vi "Next Generation.vi"(11 "cells in":bool[][](array[boolean])=[[FALSE, FALSE, TRUE, FALSE, FALSE, FALSE, FALSE, FALSE, FALSE, FALSE, FALSE, FALSE, FALSE, FALSE, FALSE, FALSE], [FALSE, FALSE, FALSE, TRUE, TRUE, FALSE, FALSE, FALSE, FALSE, FALSE, FALSE, FALSE, FALSE, FALSE, FALSE, FALSE], [FALSE, FALSE, FALSE, FALSE, FALSE, FALSE, FALSE, FALSE, FALSE, FALSE, FALSE, FALSE, FALSE, FALSE, FALSE, FALSE], [FALSE, FALSE, FALSE, FALSE, FALSE, FALSE, FALSE, FALSE, FALSE, FALSE, FALSE, FALSE, FALSE, FALSE, FALSE, FALSE], [FALSE, FALSE, FALSE, FALSE, FALSE, FALSE, FALSE, FALSE, FALSE, FALSE, FALSE, FALSE, FALSE, FALSE, FALSE, FALSE], [FALSE, FALSE, FALSE, FALSE, FALSE, FALSE, FALSE, FALSE, FALSE, FALSE, FALSE, FALSE, FALSE, FALSE, FALSE, FALSE], [FALSE, FALSE, FALSE, FALSE, FALSE, FALSE, FALSE, TRUE, FALSE, FALSE, FALSE, FALSE, FALSE, FALSE, FALSE, FALSE], [FALSE, FALSE, FALSE, FALSE, FALSE, FALSE, FALSE, FALSE, FALSE, FALSE, FALSE, FALSE, FALSE, FALSE, FALSE, FALSE], [FALSE, FALSE, FALSE, FALSE, FALSE, FALSE, FALSE, FALSE, FALSE, FALSE, FALSE, FALSE, FALSE, FALSE, FALSE, FALSE], [FALSE, FALSE, FALSE, FALSE, FALSE, FALSE, FALSE, FALSE, FALSE, FALSE, FALSE, FALSE, FALSE, TRUE, FALSE, FALSE], [FALSE, FALSE, FALSE, FALSE, FALSE, FALSE, FALSE, FALSE, FALSE, FALSE, FALSE, FALSE, TRUE, TRUE, FALSE, FALSE], [FALSE, FALSE, FALSE, FALSE, FALSE, FALSE, FALSE, FALSE, FALSE, FALSE, FALSE, FALSE, FALSE, FALSE, TRUE, FALSE], [FALSE, FALSE, FALSE, FALSE, FALSE, FALSE, FALSE, FALSE, FALSE, FALSE, FALSE, FALSE, FALSE, FALSE, FALSE, TRUE]]) -> (1 "deaths":i32, 2 "births":i32, 3 "cells out":bool[][](array[boolean])=[[FALSE, FALSE, FALSE, TRUE, FALSE, FALSE, FALSE, FALSE, FALSE, FALSE, FALSE, FALSE, FALSE, FALSE, FALSE, FALSE], [FALSE, FALSE, FALSE, TRUE, FALSE, FALSE, FALSE, FALSE, FALSE, FALSE, FALSE, FALSE, FALSE, FALSE, FALSE, FALSE], [FALSE, FALSE, FALSE, FALSE, FALSE, FALSE, FALSE, FALSE, FALSE, FALSE, FALSE, FALSE, FALSE, FALSE, FALSE, FALSE], [FALSE, FALSE, FALSE, FALSE, FALSE, FALSE, FALSE, FALSE, FALSE, FALSE, FALSE, FALSE, FALSE, FALSE, FALSE, FALSE], [FALSE, FALSE, FALSE, FALSE, FALSE, FALSE, FALSE, FALSE, FALSE, FALSE, FALSE, FALSE, FALSE, FALSE, FALSE, FALSE], [FALSE, FALSE, FALSE, FALSE, FALSE, FALSE, FALSE, FALSE, FALSE, FALSE, FALSE, FALSE, FALSE, FALSE, FALSE, FALSE], [FALSE, FALSE, FALSE, FALSE, FALSE, FALSE, FALSE, FALSE, FALSE, FALSE, FALSE, FALSE, FALSE, FALSE, FALSE, FALSE], [FALSE, FALSE, FALSE, FALSE, FALSE, FALSE, FALSE, FALSE, FALSE, FALSE, FALSE, FALSE, FALSE, FALSE, FALSE, FALSE], [FALSE, FALSE, FALSE, FALSE, FALSE, FALSE, FALSE, FALSE, FALSE, FALSE, FALSE, FALSE, FALSE, FALSE, FALSE, FALSE], [FALSE, FALSE, FALSE, FALSE, FALSE, FALSE, FALSE, FALSE, FALSE, FALSE, FALSE, FALSE, TRUE, TRUE, FALSE, FALSE], [FALSE, FALSE, FALSE, FALSE, FALSE, FALSE, FALSE, FALSE, FALSE, FALSE, FALSE, FALSE, TRUE, TRUE, TRUE, FALSE], [FALSE, FALSE, FALSE, FALSE, FALSE, FALSE, FALSE, FALSE, FALSE, FALSE, FALSE, FALSE, FALSE, TRUE, TRUE, FALSE], [FALSE, FALSE, FALSE, FALSE, FALSE, FALSE, FALSE, FALSE, FALSE, FALSE, FALSE, FALSE, FALSE, FALSE, FALSE, FALSE]])   [LabVIEW 2021, in "Game Of Life.lvlib"]
uses:
  Game Of Life.lvlib
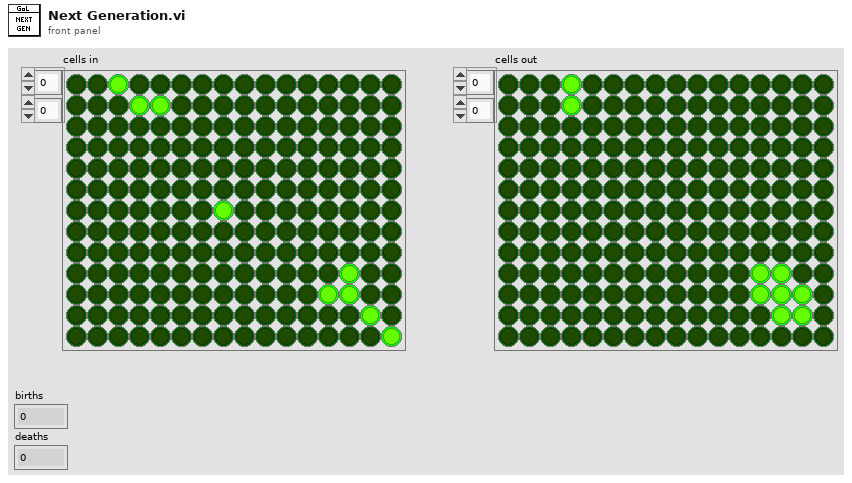
[diagram p1: front panel]
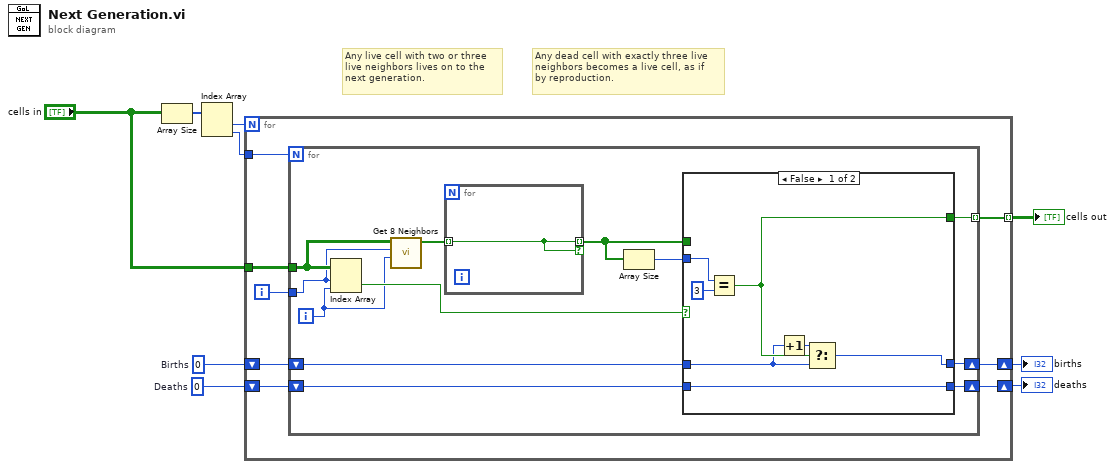
[diagram p0: block diagram]
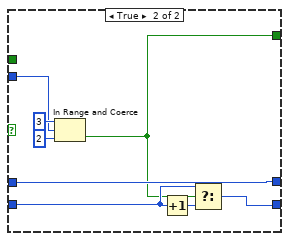
[diagram p2: hidden frame]
diagram:
  w4 = 0  # Deaths
  w5 = 0  # Births
  # "Any live cell with two or three\nlive neighbors lives on to the\nnext generation."
  # "Any dead cell with exactly three live\nneighbors becomes a live cell, as if\nby reproduction."
  n1 = Array Size(array="cells in") -> (size(s)=w9:i32[])
  n2 = Index Array(array=w9) -> (element #1=w8:i32, element #2=w7:i32)  [unwired: 2 in]
  n3 = for {
    N: w8 -> [_]
    tunnel: w7 -> [w16]
    tunnel: [w15] -> w1 mode=indexing
    shift-right: [w14] -> w6
    shift-left: w5 -> [w13]
    shift-right: [w11] -> w3
    shift-left: w4 -> [w12]
    tunnel: "cells in" -> [w10]
    i -> [w17]
    n4 = for {
      N: w16 -> [_]
      tunnel: w17 -> [w22]
      tunnel: [w29] -> w15 mode=indexing
      shift-right: [w28] -> w14
      shift-left: w13 -> [w27]
      shift-right: [w25] -> w11
      shift-left: w12 -> [w26]
      tunnel: w10 -> [w23]
      i -> [w21]
      n5 = Index Array(array=w23, index (row)=w22, index (col)=w21) -> (element=w24:bool)
      n6 = call "Get 8 Neighbors.vi"("column"=w21, "row"=w22, "cells in"=w23) -> ("cells living"=w20:bool[])  [unwired: 8 in]
      n7 = for {
        tunnel: w20 -> [w30] mode=indexing
        tunnel: [w30] -> w18 mode=indexing if=w30
      }
      n8 = Array Size(array=w18) -> (size(s)=w19:i32)
      n9 = case shown="False" w24 {
        tunnel: [w35 w39] -> w29
        tunnel: [w32 w43] -> w28
        tunnel: w27 -> [w31 w43]
        tunnel: w26 -> [w33 w41]
        tunnel: [w33 w38] -> w25
        tunnel: w19 -> [w36 w42]
        tunnel: w18 -> [_ _]
        frame False {
          n10 = Equal?(x=w36, y=3) -> (x = y?=w35:bool)
          n11 = Increment(x=w31) -> (x+1=w34:i32)
          n12 = Select(t=w34, s=w35, f=w31) -> (s? t:f=w32:i32)
        }
        frame True {
          n13 = In Range and Coerce(upper limit=3, x=w42, lower limit=2) -> (In Range?=w39:bool)  [unwired: 1 out]
          n14 = Increment(x=w41) -> (x+1=w40:i32)
          n15 = Select(t=w41, s=w39, f=w40) -> (s? t:f=w38:i32)
        }
      }
    }
  }
  "births" <- w6
  "deaths" <- w3
  "cells out" <- w1
